vi "Verduennungsgas aus Traegergas.vi"(11 "Trägergas":T1="N2" caption="Carrier Gas") -> (3 "Verdünnungsgas":T2 items=["N2", "O2"])   [LabVIEW 2020, in "Linearisierung v2.lvlib" / "SpanEinstellungen.lvlib"]
uses:
  SpanEinstellungen.lvlib
  Seiten/System Einstellungen V2/Traegergas.ctl
  Gasteiler/Gasteiler.lvlib
  Seiten/System Einstellungen V2/System Einstellungen V2.lvlib
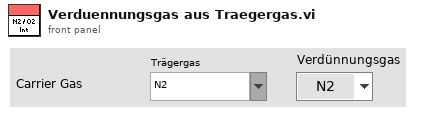
[diagram p1: front panel]
types:
  T1 = typedef "System Einstellungen V2.lvlib/Traegergas.ctl" = string
  T2 = typedef "Linearisierung v2.lvlib/Gasteiler.lvlib/Prüfgas in.ctl" = u16
  T3 = typedef "LVComboBoxStrsAndValuesArrayTypeDef.ctl" = cluster{"String":string, "Value":string}[]
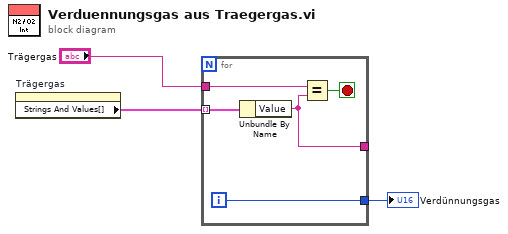
[diagram p0: block diagram]
diagram:
  n1 = property on="Trägergas" class="KombiFeld (strikt)"() -> ("Strings And Values[]"=w3:T3)  [unwired: 2 in, 2 out]
  n2 = for {
    tunnel: w3 -> [w8] mode=indexing
    tunnel: "Trägergas" -> [w7]
    tunnel: [w5] -> _
    tunnel: [w4] -> w1
    i -> [w4]
    stop <- w6 stop-if-true
    n3 = Unbundle By Name(w8) -> ("Value"=w5:string)
    n4 = Equal?(x=w7, y=w5) -> (x = y?=w6:bool)
  }
  "Verdünnungsgas" <- w1
